vi "MH_ReadPTUAndQueue.vi"() -> ()   [LabVIEW 2019]
doc: "Read Binary File opens and reads an existing file stored as a double precision array in binary form. This VI shows the simplest way to read this entire file, with the simplest error checking."
uses:
  <userlib>/MultiHarp150/T2Lib/MH_T2QMessage.ctl
panel:
  in  "buff size":i32
  out "Processing:":i32
  out "GlobalResolution":dbl
  out "Resolution":dbl
  out "NumberOfRecords":i64
  out "TTTRRecType":i64 format="%x"
  out "n_hdr_items":i32=80
  out "Version":string
  out "Magic":string
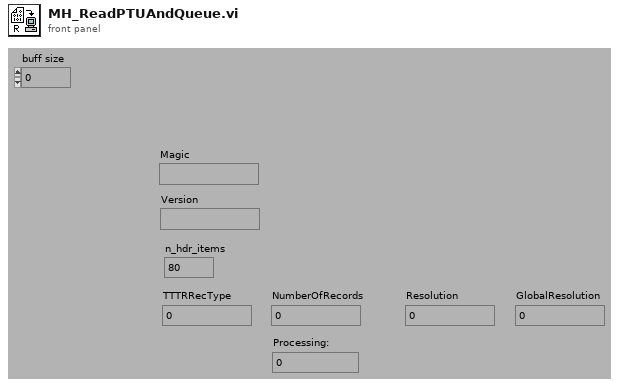
[diagram p1: front panel]
types:
  T1 = typedef "MH_T2QMessage.ctl" = cluster{"Message":string, "buffer":u32[], "Code":i32, "nactual":i32}
  T2 = cluster{"TagIdent":string, "TagIndex":i32, "TagType":i32, "TagValue":i64, "TagAuxData":string}
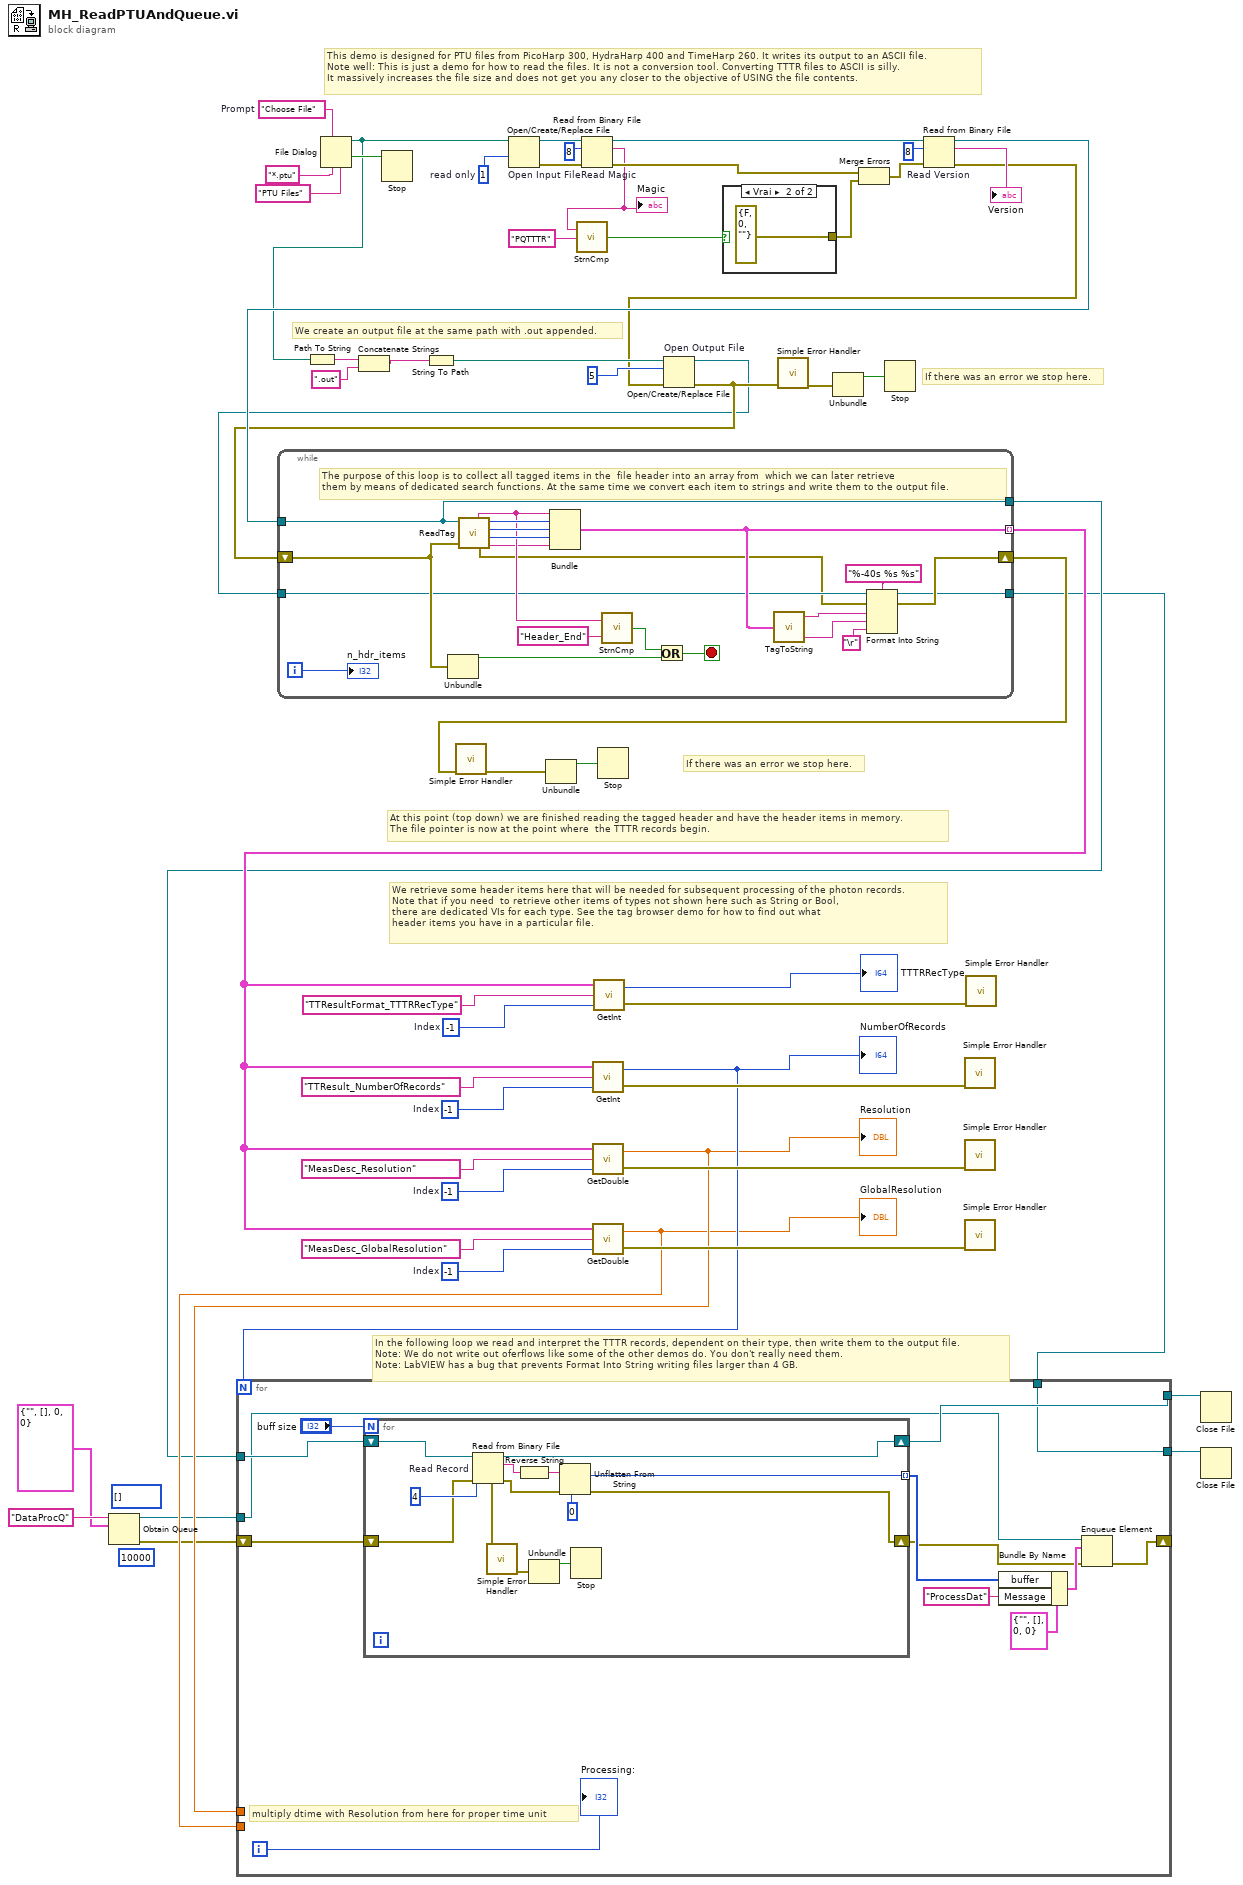
[diagram p0: block diagram]
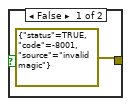
[diagram p2: hidden frame]
diagram:
  (unwired) 10000 ("timeout en ms (-1)")
  (unwired) i32[] [] ("DeltaT")
  w16 = -1  # Index
  w33 = -1  # Index
  w36 = -1  # Index
  w39 = -1  # Index
  w5 = 1  # read only
  w57 = "Choose File"  # Prompt
  # "This demo is designed for PTU files from PicoHarp 300, HydraHarp 400 and TimeHarp 260. It writes its output to an ASCII file.\nNote well: This is just a demo for how to read the files. It is not a conversion tool. Converting TTTR files to ASCII is silly.\nIt massively increases the file size and does not get you any closer to the objective of USING the file contents."
  # "In the following loop we read and interpret the TTTR records, dependent on their type, then write them to the output file.\nNote: We do not write out oferflows like some of the other demos do. You don't really need them.\nNote: LabVIEW has a bug that prevents Format Into String writing files larger than 4 GB."
  # "If there was an error we stop here."
  # "We create an output file at the same path with .out appended."
  # "If there was an error we stop here."
  # "At this point (top down) we are finished reading the tagged header and have the header items in memory.\nThe file pointer is now at the point where  the TTTR records begin."
  # "We retrieve some header items here that will be needed for subsequent processing of the photon records.\nNote that if you need  to retrieve other items of types not shown here such as String or Bool, \nthere are dedicated VIs for each type. See the tag browser demo for how to find out what \nheader items you have in a particular file."
  n1 = Obtain Queue(name (unnamed)="DataProcQ" ("nom (aucun)"), element data type=T1 {"Message"="", "buffer"=[], "Code"=0, "nactual"=0} ("ClassQueue")) -> (queue out=w1:refnum<queue>, error out=w2:errorcluster)  [unwired: 3 in, 1 out]
  n2 = File Dialog(4:"PTU Files", 6:"*.ptu", 7:w57) -> (1:w43:bool, 3:w28:path)  [unwired: 4 in, 2 out]
  n3 = Path To String(path=w28) -> (string=w27:string)
  n4 = Concatenate Strings(w27, ".out" ("string")) -> (w25:string)
  n5 = Stop(stop? (T)=w43) -> ()
  n6 = String To Path(string=w25) -> (path=w24:path)
  n7 = Open/Create/Replace File "Open Input File"(file path (use dialog)=w28, access (0:read/write)=w5) -> (refnum out=w45:refnum<file>, error out=w44:errorcluster)  [unwired: 4 in, 1 out]
  n8 = Read from Binary File "Read Magic"(8:w44, 10:8, 11:w45) -> (0:w52:errorcluster, 2:w48:string, 3:w56:refnum<file>)  [unwired: 3 in, 1 out]
  "Magic" <- w48
  n9 = call <userlib>:"StrnCmp.vi"("String 2"="PQTTTR", "String 1"=w48) -> ("equal"=w49:bool)
  n10 = case shown="Vrai" w49 {
    tunnel: [errorcluster {"status"=TRUE, "code"=-8001, "source"="invalid magic"} ("file error status 2") errorcluster {"status"=FALSE, "code"=0, "source"=""} ("file error status 2")] -> w50
    frame False {
    }
    frame True {
    }
  }
  n11 = Merge Errors(w52, w50) -> (w51:errorcluster)
  n12 = Read from Binary File "Read Version"(8:w51, 10:8, 11:w56) -> (0:w21:errorcluster, 2:→"Version":string, 3:w42:refnum<file>)  [unwired: 3 in, 1 out]
  n13 = Open/Create/Replace File "Open Output File"(file path (use dialog)=w24, error in=w21, operation (0:open)=5) -> (refnum out=w18:refnum<file>, error out=w20:errorcluster)  [unwired: 3 in, 1 out]
  n14 = while {
    shift-left: w20 -> [w79]
    shift-right: [w65] -> w31
    tunnel: w42 -> [w61]
    tunnel: [w69] -> w14 mode=indexing
    tunnel: w18 -> [w68]
    tunnel: [w62] -> w6
    tunnel: [w61] -> w9
    i -> [w75]
    stop <- w80 stop-if-true
    # "The purpose of this loop is to collect all tagged items in the  file header into an array from  which we can later retrieve \nthem by means of dedicated search functions. At the same time we convert each item to strings and write them to the output file."
    n15 = Unbundle(w79) -> ("status"=w72:bool)  [unwired: 2 out]
    n16 = call <userlib>:"ReadTag.vi"("refnum"=w61, "error in"=w79) -> ("TagIdent"=w71:string, "TagIndex"=w78:i32, "TagType"=w77:i32, "error out"=w66:errorcluster, "TagValue"=w76:i64, "TagAuxData"=w70:string)  [unwired: 3 in]
    n17 = Bundle("TagIdent"=w71, "TagIndex"=w78, "TagType"=w77, "TagValue"=w76, "TagAuxData"=w70) -> (w69:T2)  [unwired: 1 in]
    n18 = call <userlib>:"StrnCmp.vi"("String 2"="Header_End", "String 1"=w71) -> ("equal"=w73:bool)
    n19 = Or(x=w73, y=w72) -> (x .or. y?=w80:bool)
    n20 = call <userlib>:"TagToString.vi"("TagData"=w69) -> ("StrTagValue"=w63:string, "StrTagName"=w64:string)  [unwired: 2 in, 1 out]
    n21 = Format Into String(format string="%-40s %s %s", initial string=w68, error in=w66, w64, w63, "\r") -> (resulting string=w62:refnum<file>, error out=w65:errorcluster)
    "n_hdr_items" <- w75
  }
  n22 = call <vilib>:"Simple Error Handler.vi"("error in (no error)"=w31) -> ("error out"=w30:errorcluster)  [unwired: 4 in, 4 out]
  n23 = Unbundle(w30) -> ("status"=w29:bool)  [unwired: 2 out]
  n24 = call <userlib>:"GetInt.vi"("Index"=w36, "Ident"="TTResult_NumberOfRecords", "Array"=w14) -> ("error status"=w35:errorcluster, "TagValue"=w13:i64)
  "NumberOfRecords" <- w13
  n25 = call <userlib>:"GetDouble.vi"("Index"=w33, "Ident"="MeasDesc_Resolution", "Array"=w14) -> ("error status"=w32:errorcluster, "TagValue"=w11:dbl)
  "Resolution" <- w11
  n26 = call <userlib>:"GetDouble.vi"("Index"=w16, "Ident"="MeasDesc_GlobalResolution", "Array"=w14) -> ("error status"=w15:errorcluster, "TagValue"=w10:dbl)
  "GlobalResolution" <- w10
  n27 = for {
    N: w13 -> [_]
    tunnel: w11 -> [_]
    tunnel: w10 -> [_]
    tunnel: w9 -> [w93]
    tunnel: [w92] -> w8
    tunnel: [w91] -> w7
    tunnel: w6 -> [w91]
    shift-right: [w81] -> _
    shift-left: w2 -> [w89]
    tunnel: w1 -> [w83]
    i -> [w90]
    # "multiply dtime with Resolution from here for proper time unit"
    n28 = for {
      N: "buff size" -> [_]
      shift-right: [w100] -> w92
      shift-left: w93 -> [w101]
      shift-right: [w95] -> w82
      shift-left: w89 -> [w97]
      tunnel: [w94] -> w85 mode=indexing
      n29 = Read from Binary File "Read Record"(8:w97, 10:4, 11:w101) -> (0:w96:errorcluster, 2:w104:string, 3:w100:refnum<file>)  [unwired: 3 in, 1 out]
      n30 = call <vilib>:"Simple Error Handler.vi"("error in (no error)"=w96) -> ("error out"=w99:errorcluster)  [unwired: 4 in, 4 out]
      n31 = Reverse String(1:w104) -> (0:w105:string)
      n32 = Unbundle(w99) -> ("status"=w98:bool)  [unwired: 2 out]
      n33 = Unflatten From String(type=u32 0, binary string=w105, error in (no error)=w96) -> (value=w94:u32, error out=w95:errorcluster)  [unwired: 2 in, 1 out]
      n34 = Stop(stop? (T)=w98) -> ()
    }
    n35 = Bundle By Name(cluster=T1 {"Message"="", "buffer"=[], "Code"=0, "nactual"=0} ("ClassQueue"), "buffer"=w85, "Message"="ProcessDat") -> (w84:T1)
    n36 = Enqueue Element(queue=w83, element=w84, error in (no error)=w82) -> (error out=w81:errorcluster)  [unwired: 1 in, 2 out]
    "Processing:" <- w90
  }
  n37 = call <userlib>:"GetInt.vi"("Index"=w39, "Ident"="TTResultFormat_TTTRRecType", "Array"=w14) -> ("error status"=w38:errorcluster, "TagValue"=→"TTTRRecType":i64)
  n38 = Stop(stop? (T)=w29) -> ()
  n39 = call <vilib>:"Simple Error Handler.vi"("error in (no error)"=w20) -> ("error out"=w19:errorcluster)  [unwired: 4 in, 4 out]
  n40 = Unbundle(w19) -> ("status"=w22:bool)  [unwired: 2 out]
  n41 = Stop(stop? (T)=w22) -> ()
  n42 = call <vilib>:"Simple Error Handler.vi"("error in (no error)"=w35) -> ()  [unwired: 4 in, 5 out]
  n43 = call <vilib>:"Simple Error Handler.vi"("error in (no error)"=w32) -> ()  [unwired: 4 in, 5 out]
  n44 = call <vilib>:"Simple Error Handler.vi"("error in (no error)"=w15) -> ()  [unwired: 4 in, 5 out]
  n45 = call <vilib>:"Simple Error Handler.vi"("error in (no error)"=w38) -> ()  [unwired: 4 in, 5 out]
  n46 = Close File(refnum=w8) -> ()  [unwired: 1 in, 2 out]
  n47 = Close File(refnum=w7) -> ()  [unwired: 1 in, 2 out]
